vi "Read Batch Profiles All.vi"(0 "Device ID (0)":i32, 1 "Timeout ms (5000)":u32=5000, 5 "Read Batch Profile Req":T3 {"Batch Pos" items=["CURRENT"=0, "SPECIFY"=2, "COMMITED"=3, "NEWEST PROFILE"=4]}, 7 "Read Profile Cnt":u32=1000, 11 "error in (no error)":errorcluster {"code" format="%.0x"}) -> (2 "Timeout ?":bool, 3 "Profile Info":T2, 4 "Device ID out":i32, 6 "Header Array":u32[][](array[numeric]), 8 "Height Profile Array":dbl[][](array[numeric]), 10 "Brightness Profile Array":u16[][](array[numeric]), 14 "Read Batch Profile Rsp":T1, 15 "error out":errorcluster {"code" format="%.0x"})   [LabVIEW 2010, in "KEYENCE LJ-X8000A.lvlib"]
doc: "This function gets all batch profile data when bacth measurement is ON.\nThe height and brightness profile data are each stored in a simple array.\nThe height profile is in units of mm."
uses:
  KEYENCE LJ-X8000A.lvlib
  Clusters/Read Batch Profile Req.ctl
  Constants/Batch Pos.ctl
  Clusters/Profile Info.ctl
  Clusters/Read Batch Profile Rsp.ctl
  Clusters/Read Batch Profile Req for all read.ctl
panel:
  out "read loop count":i32
  out "Process Time ms":u32
  # "(c) 2019 KEYENCE CORPORATION.  ALL RIGHTS RESERVED."
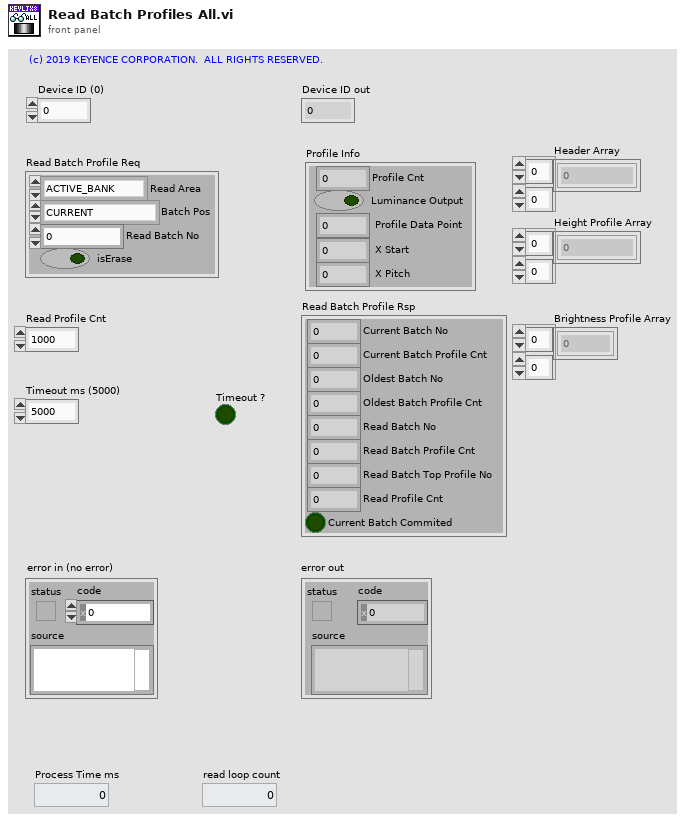
[diagram p1: front panel]
types:
  T1 = typedef "KEYENCE LJ-X8000A.lvlib/Read Batch Profile Rsp.ctl" = cluster{"Current Batch No":u32, "Current Batch Profile Cnt":u32, "Oldest Batch No":u32, "Oldest Batch Profile Cnt":u32, "Read Batch No":u32, "Read Batch Profile Cnt":u32, "Read Batch Top Profile No":u32, "Read Profile Cnt":u32, "Current Batch Commited":bool}
  T2 = typedef "KEYENCE LJ-X8000A.lvlib/Profile Info.ctl" = cluster{"Profile Cnt":u8, "Luminance Output":bool, " Profile Data Point":u16, " X Start":i32, " X Pitch":i32}
  T3 = typedef "KEYENCE LJ-X8000A.lvlib/Read Batch Profile Req for all read.ctl" = cluster{"Read Area":enum8{"ACTIVE_BANK", "INACTIVE_BANK"}, "Batch Pos":T4, "Read Batch No":u32, "isErase":bool}
  T4 = typedef "KEYENCE LJ-X8000A.lvlib/Batch Pos.ctl" = u8
  T5 = typedef "KEYENCE LJ-X8000A.lvlib/Read Batch Profile Req.ctl" = cluster{"Read Area":enum8{"ACTIVE_BANK", "INACTIVE_BANK"}, "Batch Pos":T4, "Read Batch No":u32, "Read Profile No.":u32, "Read Profile Cnt":u8, "isErase":bool}
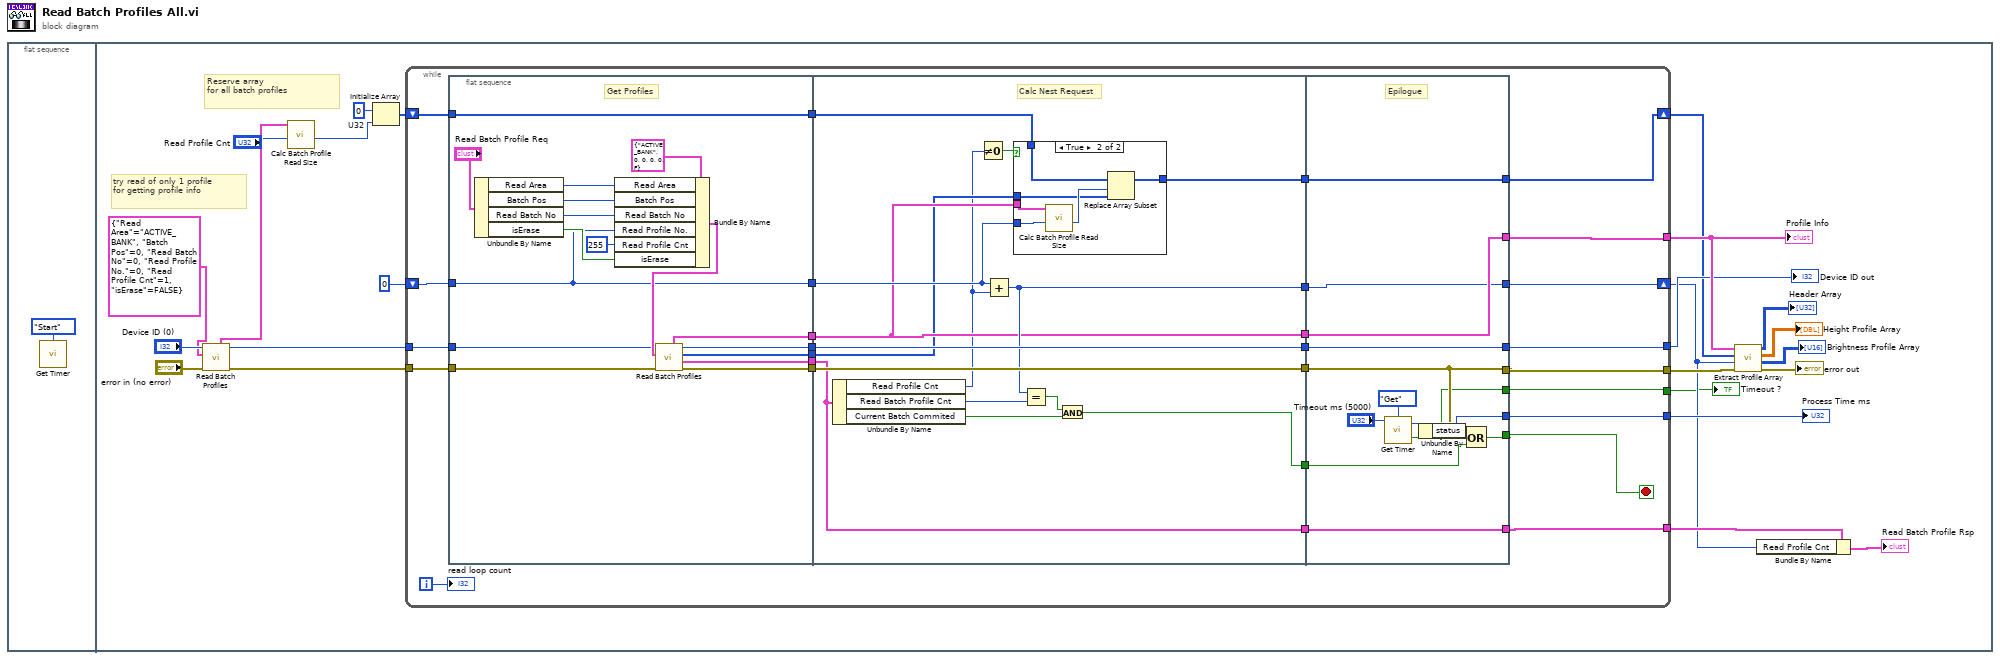
[diagram p0: block diagram]
diagram:
  n1 = flat-sequence {
    frame #0 {
      n2 = call "Get Timer.vi"("Mode"=enum8{"Start", "Get"}."Start") -> ()  [unwired: 3 in, 2 out]
    }
    frame #1 {
      w18 = u32 0  # U32
      # "Reserve array\nfor all batch profiles"
      # "try read of only 1 profile \nfor getting profile info"
      n3 = call "Read Batch Profiles.vi"("error in (no error)"="error in (no error)", "Read Batch Profile Req"=T5 {"Read Area"=enum."ACTIVE_BANK", "Batch Pos"=0, "Read Batch No"=0, "Read Profile No."=0, "Read Profile Cnt"=1, "isErase"=FALSE}, "Device ID (0)"="Device ID (0)") -> ("error out"=w17:errorcluster, "Device ID out"=w16:i32, "Profile Info"=w20:T2)  [unwired: 4 in, 2 out]
      n4 = call "Calc Batch Profile Read Size.vi"("Read Profile Cnt"="Read Profile Cnt", "Profile Info"=w20) -> ("Required Size(DWORD)"=w14:u32)  [unwired: 8 in, 1 out]
      n5 = Initialize Array(w18, w14) -> (w15:u32[])
      n6 = while {
        shift-right: [w38] -> w3
        shift-left: u32 0 ("Read Profile No.") -> [w51]
        tunnel: [w52] -> w24
        tunnel: [w50] -> w13
        tunnel: [w49] -> w11
        tunnel: [w48] -> w4
        tunnel: w17 -> [w35]
        tunnel: w16 -> [w36]
        shift-right: [w30] -> w10
        shift-left: w15 -> [w34]
        tunnel: [w28] -> w6
        tunnel: [w26] -> w2
        i -> [w27]
        stop <- w53 stop-if-true
        n7 = flat-sequence {
          tunnel: [w55] -> w47
          tunnel: w51 -> [w61]
          tunnel: [w64] -> w45
          tunnel: [w63] -> w43
          tunnel: [w62] -> w41
          tunnel: [w61] -> w40
          tunnel: w36 -> [w59]
          tunnel: w35 -> [w54]
          tunnel: w34 -> [w58]
          tunnel: [w58] -> w33
          tunnel: [w57] -> w32
          tunnel: w47 -> [w85]
          tunnel: [w85] -> w46
          tunnel: w45 -> [w76]
          tunnel: [w76] -> w44
          tunnel: w43 -> [w84]
          tunnel: [w84] -> w42
          tunnel: w41 -> [w72]
          tunnel: w40 -> [w77]
          tunnel: [w83] -> w39
          tunnel: [w79] -> w37
          tunnel: w33 -> [w75]
          tunnel: w32 -> [w74]
          tunnel: [w73] -> w31
          tunnel: [w72] -> w29
          tunnel: w46 -> [w101]
          tunnel: [w105] -> w53
          tunnel: [w104] -> w52
          tunnel: w44 -> [w103]
          tunnel: [w103] -> w50
          tunnel: [w102] -> w49
          tunnel: w42 -> [w102]
          tunnel: [w101] -> w48
          tunnel: w39 -> [w100]
          tunnel: [w100] -> w38
          tunnel: w37 -> [w99]
          tunnel: w31 -> [w98]
          tunnel: [w98] -> w30
          tunnel: w29 -> [w97]
          tunnel: [w97] -> w28
          tunnel: [w94] -> w26
          frame #0 {
            # "Get Profiles"
            n8 = Unbundle By Name("Read Batch Profile Req") -> ("Read Area"=w66:enum8{"ACTIVE_BANK", "INACTIVE_BANK"}, "Batch Pos"=w60:T4, "Read Batch No"=w67:u32, "isErase"=w68:bool)
            n9 = Bundle By Name(cluster=T5 {"Read Area"=enum."ACTIVE_BANK", "Batch Pos"=0, "Read Batch No"=0, "Read Profile No."=0, "Read Profile Cnt"=0, "isErase"=FALSE} ("Read Batch Profile Req"), "Read Area"=w66, "Batch Pos"=w60, "Read Batch No"=w67, "Read Profile No."=w61, "Read Profile Cnt"=u8 255, "isErase"=w68) -> (w65:T5)
            n10 = call "Read Batch Profiles.vi"("error in (no error)"=w54, "Read Batch Profile Req"=w65, "Device ID (0)"=w59) -> ("error out"=w55:errorcluster, "Read Batch Profile Rsp"=w62:T1, "Profile Data"=w57:u32[], "Device ID out"=w63:i32, "Profile Info"=w64:T2)  [unwired: 4 in]
          }
          frame #1 {
            # "Calc Nest Request"
            n11 = Unbundle By Name(w72) -> ("Read Profile Cnt"=w71:u32, "Read Batch Profile Cnt"=w82:u32, "Current Batch Commited"=w81:bool)
            n12 = Not Equal To 0?(x=w71) -> (x != 0?=w78:bool)
            n13 = Add(x=w77, y=w71) -> (x+y=w83:u32)
            n14 = case shown="True" w78 {
              tunnel: w77 -> [_ w92]
              tunnel: w76 -> [_ w91]
              tunnel: w75 -> [w86 w90]
              tunnel: w74 -> [_ w88]
              tunnel: [w86 w87] -> w73
              frame False {
              }
              frame True {
                n15 = call "Calc Batch Profile Read Size.vi"("Read Profile Cnt"=w92, "Profile Info"=w91) -> ("Required Size(DWORD)"=w89:u32)  [unwired: 8 in, 1 out]
                n16 = Replace Array Subset(array=w90, new element=w88, index=w89) -> (w87:u32[])
              }
            }
            n17 = Equal?(x=w83, y=w82) -> (x = y?=w80:bool)
            n18 = And(x=w80, y=w81) -> (x .and. y?=w79:bool)
          }
          frame #2 {
            # "Epilogue"
            n19 = call "Get Timer.vi"("Mode"=enum8{"Start", "Get"}."Get", "Timeout(ms)"="Timeout ms (5000)") -> ("Timeout ?"=w94:bool, "Time(ms)"=w104:u32)  [unwired: 2 in]
            n20 = Unbundle By Name(w101) -> ("status"=w93:bool)
            n21 = Compound Arithmetic op=OR ("複合演算")(w93, w94, w99) -> (w105:bool)
          }
        }
        "read loop count" <- w27
      }
      "Process Time ms" <- w24
      "Profile Info" <- w13
      "Device ID out" <- w11
      "Timeout ?" <- w2
      n22 = call "Extract Profile Array.vi"("error in (no error)"=w4, "Profile Cnt"=w3, "Profile Data"=w10, "Profile Info"=w13) -> ("error out"=→"error out":errorcluster, "Luminance Profile Array"=→"Brightness Profile Array":u16[][], "Height Profile Array"=→"Height Profile Array":dbl[][], "Header Array"=→"Header Array":u32[][])  [unwired: 4 in]
      n23 = Bundle By Name(cluster=w6, "Read Profile Cnt"=w3) -> (→"Read Batch Profile Rsp":T1)
    }
  }
